vi "Get Transfer Group Names.vi"(11 "UDP Transceiver in":refnum<class "UDP Transceiver.lvclass">) -> (2 "Transfer Group names":string[](array[string]), 3 "UDP Transceiver out":refnum<class "UDP Transceiver.lvclass">)   [LabVIEW 2017, in "UDP Transceiver.lvlib" / "UDP Transceiver.lvclass"]
uses:
  UDP Transceiver.lvclass
  UDP Transceiver.lvclass/UDP Transceiver.ctl
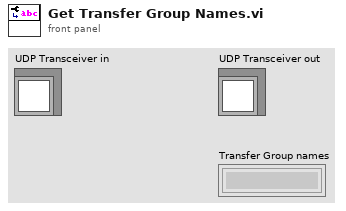
[diagram p1: front panel]
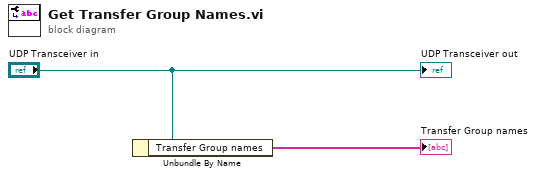
[diagram p0: block diagram]
diagram:
  n1 = Unbundle By Name("UDP Transceiver in") -> ("Transfer Group names"=→"Transfer Group names":string[])
  "UDP Transceiver out" <- "UDP Transceiver in"
